vi "Download_Scale.vi"(7 "ScaledValue":T1=1000000 items=["Bytes"=1, "KB"=1000, "MB"=1000000, "GB"=1000000000], 11 "DownloadStats In":T2) -> (3 "RunningStats":T2)   [LabVIEW 2018, in "LabVIEWHTTPClient_NET.lvlib" / "HttpContent.lvclass"]
uses:
  HttpContent.lvclass
  Types/DownloadStats_Cluster.ctl
  Types/ScaledValue_ring.ctl
  LabVIEWHTTPClient_NET/LabVIEWHTTPClient_NET.lvlib
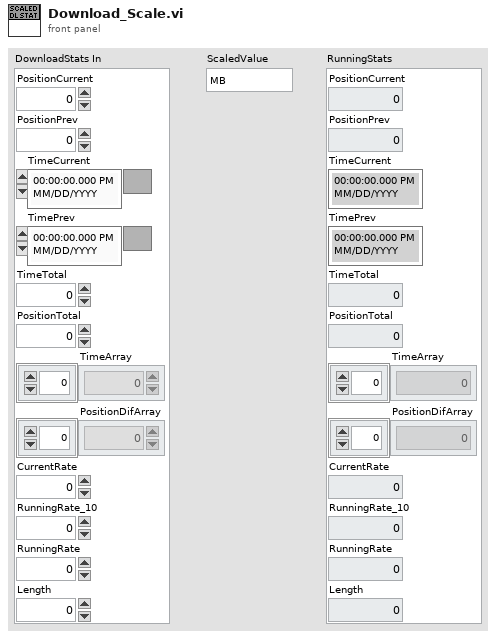
[diagram p1: front panel]
types:
  T1 = typedef "LabVIEWHTTPClient_NET.lvlib/ScaledValue_ring.ctl" = u64
  T2 = typedef "LabVIEWHTTPClient_NET.lvlib/DownloadStats_Cluster.ctl" = cluster{"PositionCurrent":dbl, "PositionPrev":dbl, "TimeCurrent":timestamp, "TimePrev":timestamp, "TimeTotal":dbl, "PositionTotal":dbl, "TimeArray":dbl[], "PositionDifArray":dbl[], "CurrentRate":dbl, "RunningRate_10":dbl, "RunningRate":dbl, "Length":dbl}
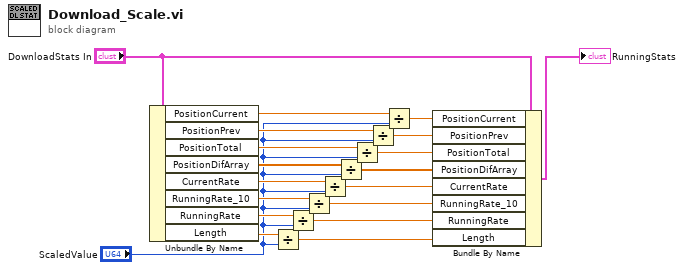
[diagram p0: block diagram]
diagram:
  n1 = Unbundle By Name("DownloadStats In") -> ("PositionCurrent"=w19:dbl, "PositionPrev"=w18:dbl, "PositionTotal"=w17:dbl, "PositionDifArray"=w16:dbl[], "CurrentRate"=w4:dbl, "RunningRate_10"=w15:dbl, "RunningRate"=w14:dbl, "Length"=w3:dbl)
  n2 = Divide(x=w3, y="ScaledValue") -> (x/y=w1:dbl)
  n3 = Divide(x=w14, y="ScaledValue") -> (x/y=w11:dbl)
  n4 = Divide(x=w15, y="ScaledValue") -> (x/y=w10:dbl)
  n5 = Divide(x=w4, y="ScaledValue") -> (x/y=w9:dbl)
  n6 = Divide(x=w16, y="ScaledValue") -> (x/y=w8:dbl[])
  n7 = Divide(x=w17, y="ScaledValue") -> (x/y=w7:dbl)
  n8 = Divide(x=w18, y="ScaledValue") -> (x/y=w6:dbl)
  n9 = Divide(x=w19, y="ScaledValue") -> (x/y=w5:dbl)
  n10 = Bundle By Name(cluster="DownloadStats In", "PositionCurrent"=w5, "PositionPrev"=w6, "PositionTotal"=w7, "PositionDifArray"=w8, "CurrentRate"=w9, "RunningRate_10"=w10, "RunningRate"=w11, "Length"=w1) -> (→"RunningStats":T2)
